vi "SubpanelGuiTemplate.vi"() -> ()   [LabVIEW 2016]
uses:
  <vilib>/Utility/miscctls.llb/LVRowAndColumnUnsignedTypeDef.ctl
  Controls/Messages/DAQControl.ctl
panel:
  in  "Average":bool
  in  "Device":tag
  in  "Add Channel":bool
  in  "Channel":string
  in  "Channel Name":string
  in  "Save Config":bool
  in  "Load Config":bool
  in  "Measurement Rate (Hz)":dbl=2.0
  in  "Average Samples":i32=10
  in  "Stop DAQ":bool
  in  "Start DAQ":bool
  in  "Thermocouple Channels":i32(listbox)
  in  "Remove":bool
  in  "Add":bool
  in  "Control Thermocouple Channels":i32(listbox)
  out "Temperature Profile":cluster{"X":dbl[], "Y":dbl[]}[](graph)
  in  "Name":string="Cycle 1"
  in  "Clear Temps":bool
  in  "Remove Temp":bool
  in  "Add Temp":bool
  in  "Duration":timestamp caption="Duration\n(Hours)" format="%<%H:%M:%S>T"
  in  "Temp":dbl=25.0 caption="Temperature\n(Celsius)"
  in  "Temp Profile List":i32(listbox)=-1
  in  "SaveProfile":bool
  in  "LoadProfile":bool
  in  "Operational Low":dbl=-35.0
  in  "Operational High":dbl=65.0
  in  "Survival Low":dbl=-40.0
  in  "Survival High":dbl=70.0
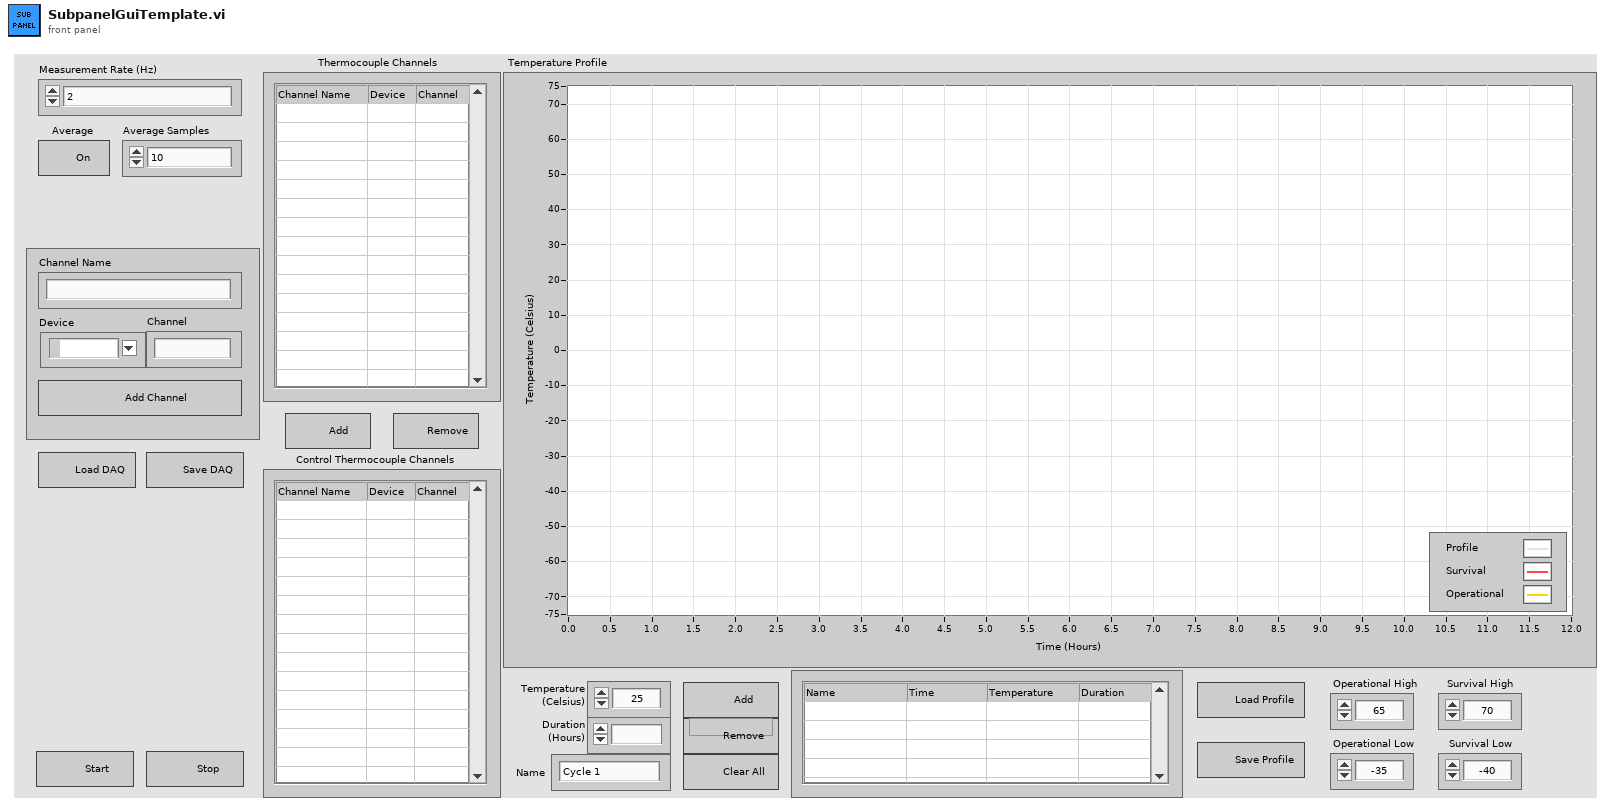
[diagram p1: front panel]
types:
  T1 = typedef "LVRowAndColumnUnsignedTypeDef.ctl" = cluster{"Row":u32, "Column":u32}
  T2 = cluster{"Error":errorcluster, "ChannelList":cluster{"Name":string, "Device":tag, "Channel":string}[], "SampleFreq":dbl, "AvgSamples":i32, "Average":bool, "SampleRate":dbl, "MaxHours":dbl, "TempProfile":dbl[][], "DurationString":string[], "Profile":cluster{"Name":string, "Temperature":string, "Duration":dbl, "Survival High":dbl, "Operational High":dbl, "Operational Low":dbl, "Survival Low":dbl}[], "TempProfileName":string[]}
  T3 = cluster{"Name":string, "Device":tag, "Channel":string}[]
  T4 = cluster{"Name":string, "Device":tag, "Channel":string}
  T5 = typedef "DAQControl.ctl" = cluster{"Timestamp":string, "Timestamp In Seconds":dbl, "DAQ Settings":cluster{"Frequency":dbl, "Averaging":bool, "Average Samples":i32}, "TC Channels":cluster{"Name":string, "Device":string, "Channel":string}[], "Control TCs":string[], "Profile":cluster{"Name":string, "Duration":string, "Temperature":dbl, "Survival High":dbl, "Operational High":dbl, "Operational Low":dbl, "Survival Low":dbl}[], "State":bool}
  T6 = typedef "LVRectTypeDef.ctl" = cluster{"Left":i16, "Top":i16, "Right":i16, "Bottom":i16}
  T7 = cluster{"Channel Name":string, "Device":tag, "Channel":string}
  T8 = cluster{"Channel Name":string, "Device":tag, "Channel":string}[]
  T9 = cluster{"Name":string, "Temperature":string, "Duration":dbl, "Survival High":dbl, "Operational High":dbl, "Operational Low":dbl, "Survival Low":dbl}[]
  T10 = cluster{"SampleFreq":dbl, "Average":bool, "AvgSamples":i32}
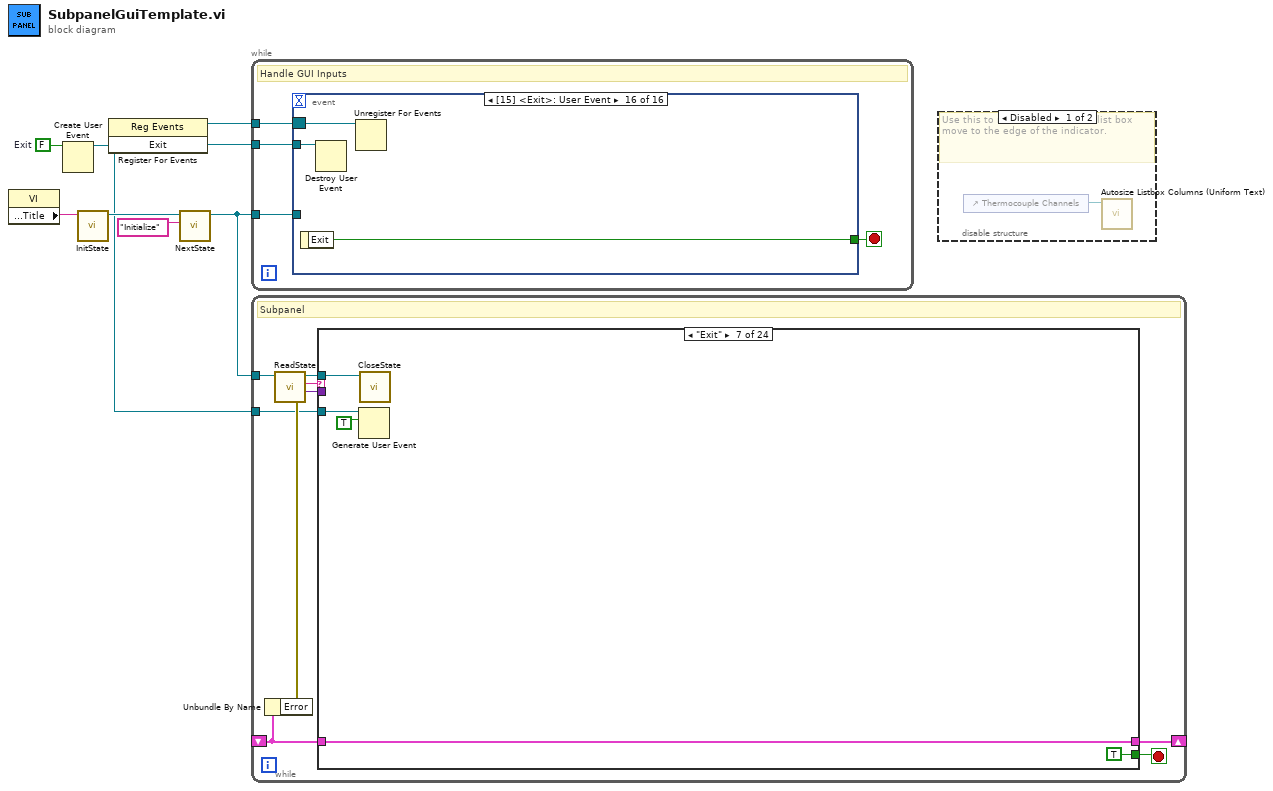
[diagram p0: block diagram]
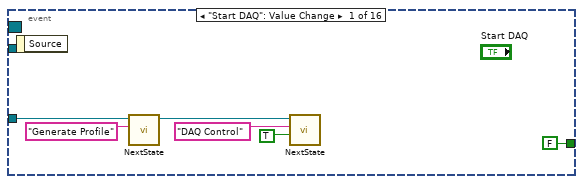
[diagram p3: hidden frame]
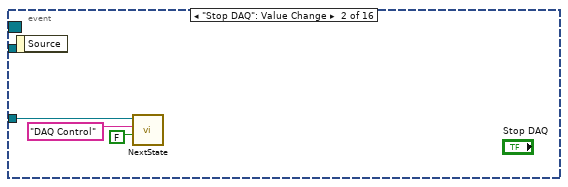
[diagram p4: hidden frame]
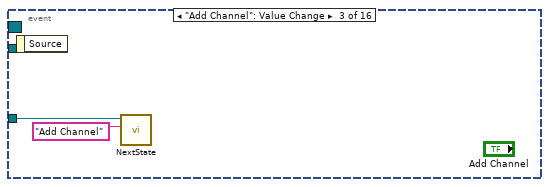
[diagram p5: hidden frame]
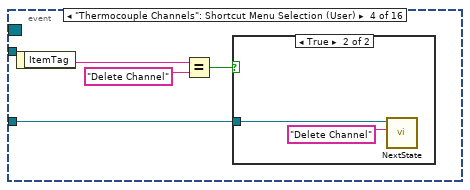
[diagram p6: hidden frame]
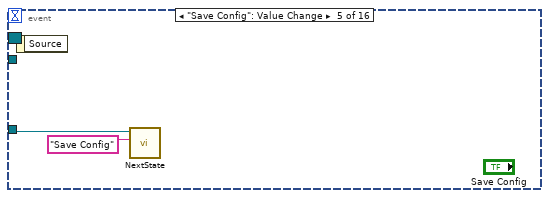
[diagram p8: hidden frame]
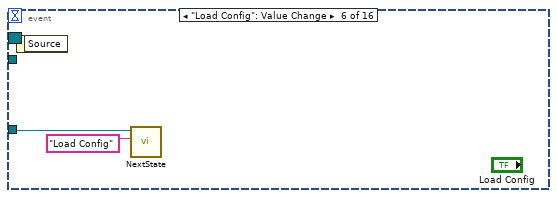
[diagram p9: hidden frame]
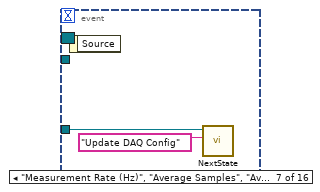
[diagram p10: hidden frame]
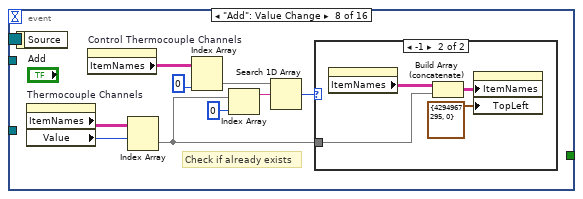
[diagram p11: hidden frame]
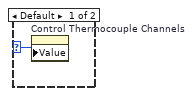
[diagram p12: hidden frame]
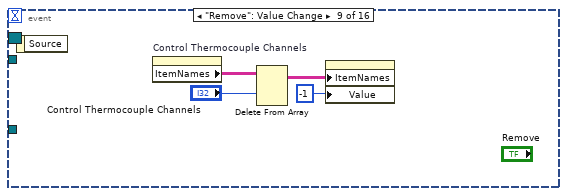
[diagram p13: hidden frame]
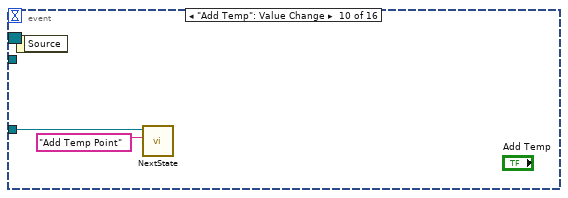
[diagram p14: hidden frame]
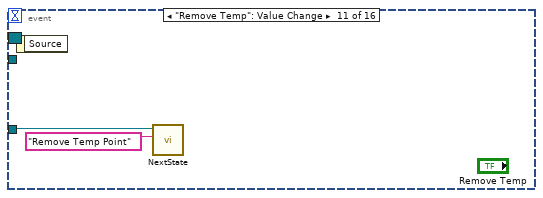
[diagram p15: hidden frame]
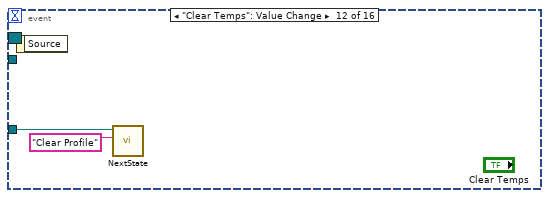
[diagram p16: hidden frame]
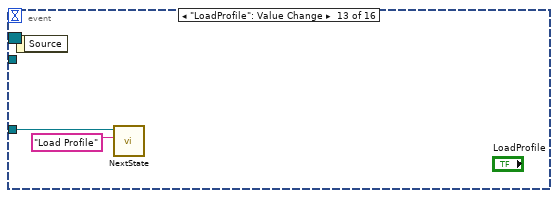
[diagram p17: hidden frame]
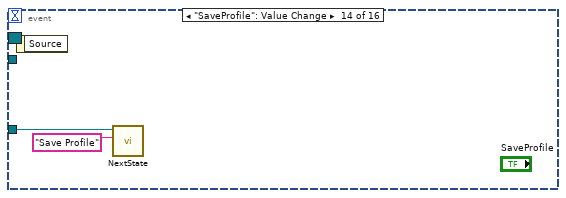
[diagram p18: hidden frame]
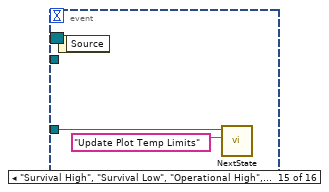
[diagram p19: hidden frame]
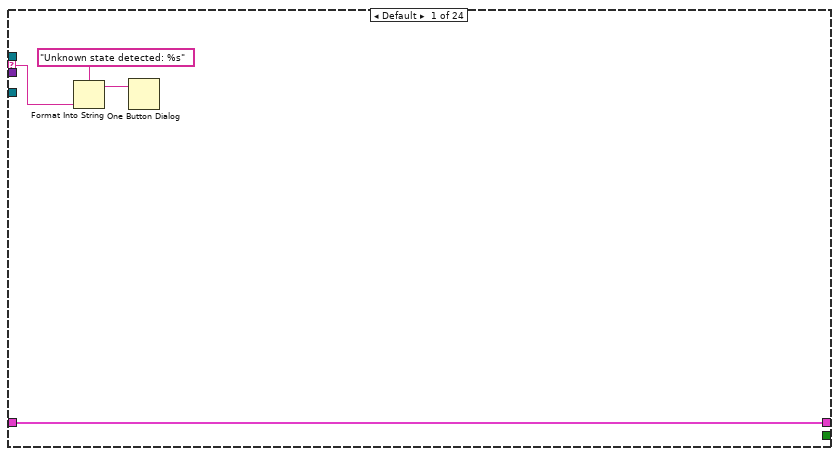
[diagram p20: hidden frame]
diagram:
  w3 = FALSE  # Exit
  n1 = property class="VI"() -> ("Front Panel.Title"=w4:string)  [unwired: 2 in, 2 out]
  n2 = Create User Event(user event datatype=w3) -> (user event=w1:refnum<user-event>)  [unwired: 1 in, 1 out]
  n3 = call "InitState.vi"("Name"=w4) -> ("Queue Out"=w7:refnum<queue>)  [unwired: 8 in, 1 out]
  n4 = register-events(w1) -> (reference out=w2:refnum<event-registration>)  [unwired: 2 in, 1 out]
  n5 = call "NextState.vi"("State"="Initialize" ("element"), "Queue In"=w7) -> ("Queue Out"=w5:refnum<queue>)  [unwired: 8 in, 1 out]
  n6 = while {
    tunnel: w5 -> [w11]
    tunnel: w2 -> [w9]
    tunnel: w1 -> [w8]
    stop <- w10 stop-if-true
    # "Handle GUI Inputs"
    n7 = event shown="[15] <Exit>: User Event" {
      selector: w9 -> [_ _ _ _ _ _ _ _ _ _ _ _ _ _ _ w67]
      dyn-events: _ -> [_ _ _ _ _ _ _ _ _ _ _ _ _ _ _ _]
      timeout: _ -> [_ _ _ _ _ _ _ _ _ _ _ _ _ _ _ _]
      tunnel: w11 -> [w15 w20 w21 w23 w29 w31 w34 _ _ w53 w56 w58 w59 w61 w63 _]
      tunnel: [FALSE _ _ _ _ _ _ _ _ _ _ _ _ _ _ w66] -> w10
      tunnel: w8 -> [_ _ _ _ _ _ _ _ _ _ _ _ _ _ _ w65]
      event "Start DAQ": Value Change {
        n8 = event-data() -> ()  [unwired: 1 in, 1 out]
        n9 = call "NextState.vi"("State"="Generate Profile" ("element"), "Queue In"=w15) -> ("Queue Out"=w14:refnum<queue>)  [unwired: 8 in, 1 out]
        n10 = call "NextState.vi"("Data"=TRUE, "State"="DAQ Control" ("element"), "Queue In"=w14) -> ()  [unwired: 7 in, 2 out]
      }
      event "Stop DAQ": Value Change {
        n11 = event-data() -> ()  [unwired: 1 in, 1 out]
        n12 = call "NextState.vi"("Data"=FALSE, "State"="DAQ Control" ("element"), "Queue In"=w20) -> ()  [unwired: 7 in, 2 out]
      }
      event "Add Channel": Value Change {
        n13 = event-data() -> ()  [unwired: 1 in, 1 out]
        n14 = call "NextState.vi"("State"="Add Channel" ("element"), "Queue In"=w21) -> ()  [unwired: 8 in, 2 out]
      }
      event "Thermocouple Channels": Shortcut Menu Selection (User) {
        n15 = event-data() -> ("ItemTag"=w26:string)  [unwired: 1 in]
        n16 = Equal?(x=w26, y="Delete Channel") -> (x = y?=w24:bool)
        n17 = case shown="True" w24 {
          tunnel: w23 -> [_ w27]
          frame False {
          }
          frame True {
            n18 = call "NextState.vi"("State"="Delete Channel" ("element"), "Queue In"=w27) -> ()  [unwired: 8 in, 2 out]
          }
        }
      }
      event "Save Config": Value Change {
        n19 = event-data() -> ()  [unwired: 1 in, 1 out]
        n20 = call "NextState.vi"("State"="Save Config" ("element"), "Queue In"=w29) -> ()  [unwired: 8 in, 2 out]
      }
      event "Load Config": Value Change {
        n21 = event-data() -> ()  [unwired: 1 in, 1 out]
        n22 = call "NextState.vi"("State"="Load Config" ("element"), "Queue In"=w31) -> ()  [unwired: 8 in, 2 out]
      }
      event "Measurement Rate (Hz)", "Average Samples", "Average": Value Change {
        n23 = event-data() -> ()  [unwired: 1 in, 1 out]
        n24 = call "NextState.vi"("State"="Update DAQ Config" ("element"), "Queue In"=w34) -> ()  [unwired: 8 in, 2 out]
      }
      event "Add": Value Change {
        # "Check if already exists"
        n25 = event-data() -> ()  [unwired: 1 in, 1 out]
        n26 = property on="Thermocouple Channels" class="MCListbox (strict)"() -> ("ItemNames"=w43:string[][], "Value"=w42:i32)  [unwired: 2 in, 2 out]
        n27 = property on="Control Thermocouple Channels" class="MCListbox (strict)"() -> ("ItemNames"=w41:string[][])  [unwired: 2 in, 2 out]
        n28 = Index Array(array=w43, index (row)=w42) -> (element=w35:string[])  [unwired: 1 in]
        n29 = Index Array(array=w41, index (col)=0 ("disabled index (col)")) -> (element=w37:string[])  [unwired: 1 in]
        n30 = Index Array(array=w35, index=0) -> (element=w38:string)
        n31 = Search 1D Array(1D array=w37, element=w38) -> (index of element=w36:i32)  [unwired: 1 in]
        n32 = case shown="-1" w36 {
          selector: w36 -> [w44 _]
          tunnel: w35 -> [_ w46]
          frame Default {
            n33 = property on="Control Thermocouple Channels" class="MCListbox (strict)"("Value"=w44) -> ()  [unwired: 2 in, 2 out]
          }
          frame -1 {
            n34 = property on="Control Thermocouple Channels" class="MCListbox (strict)"() -> ("ItemNames"=w48:string[][])  [unwired: 2 in, 2 out]
            n35 = Build Array (concatenate)(w48, w46) -> (w47:string[][])
            n36 = property on="Control Thermocouple Channels" class="MCListbox (strict)"("ItemNames"=w47, "TopLeft"=T1 {"Row"=4294967295, "Column"=0} ("Top Left Visible Cell")) -> ()  [unwired: 2 in, 2 out]
          }
        }
      }
      event "Remove": Value Change {
        n37 = event-data() -> ()  [unwired: 1 in, 1 out]
        n38 = property on="Control Thermocouple Channels" class="MCListbox (strict)"() -> ("ItemNames"=w52:string[][])  [unwired: 2 in, 2 out]
        n39 = Delete From Array(array=w52, index (row)="Control Thermocouple Channels") -> (array with subset deleted=w51:string[][])  [unwired: 2 in, 1 out]
        n40 = property on="Control Thermocouple Channels" class="MCListbox (strict)"("ItemNames"=w51, "Value"=-1 ("Control Thermocouple Channels")) -> ()  [unwired: 2 in, 2 out]
      }
      event "Add Temp": Value Change {
        n41 = event-data() -> ()  [unwired: 1 in, 1 out]
        n42 = call "NextState.vi"("State"="Add Temp Point" ("element"), "Queue In"=w53) -> ()  [unwired: 8 in, 2 out]
      }
      event "Remove Temp": Value Change {
        n43 = event-data() -> ()  [unwired: 1 in, 1 out]
        n44 = call "NextState.vi"("State"="Remove Temp Point" ("element"), "Queue In"=w56) -> ()  [unwired: 8 in, 2 out]
      }
      event "Clear Temps": Value Change {
        n45 = event-data() -> ()  [unwired: 1 in, 1 out]
        n46 = call "NextState.vi"("State"="Clear Profile" ("element"), "Queue In"=w58) -> ()  [unwired: 8 in, 2 out]
      }
      event "LoadProfile": Value Change {
        n47 = event-data() -> ()  [unwired: 1 in, 1 out]
        n48 = call "NextState.vi"("State"="Load Profile" ("element"), "Queue In"=w59) -> ()  [unwired: 8 in, 2 out]
      }
      event "SaveProfile": Value Change {
        n49 = event-data() -> ()  [unwired: 1 in, 1 out]
        n50 = call "NextState.vi"("State"="Save Profile" ("element"), "Queue In"=w61) -> ()  [unwired: 8 in, 2 out]
      }
      event "Survival High", "Survival Low", "Operational High", "Operational Low": Value Change {
        n51 = event-data() -> ()  [unwired: 1 in, 1 out]
        n52 = call "NextState.vi"("State"="Update Plot Temp Limits" ("element"), "Queue In"=w63) -> ()  [unwired: 8 in, 2 out]
      }
      event User Event {
        n53 = event-data() -> ("Exit"=w66:bool)  [unwired: 1 in]
        n54 = Destroy User Event(user event=w65) -> ()  [unwired: 1 in, 1 out]
        n55 = Unregister For Events(event registration refnum=w67) -> ()  [unwired: 1 in, 1 out]
      }
    }
  }
  n56 = while {
    tunnel: w5 -> [w74]
    shift-right: [w76] -> _
    shift-left: _ -> [w70]
    tunnel: w1 -> [w68]
    stop <- w75 stop-if-true
    # "Subpanel"
    n57 = Unbundle By Name(w70) -> ("Error"=w69:errorcluster)
    n58 = call "ReadState.vi"("Error In"=w69, "Queue In"=w74) -> ("Data"=w71:variant, "State"=w72:string, "Queue Out"=w73:refnum<queue>)  [unwired: 6 in, 1 out]
    n59 = case shown="\"Exit\"" w72 {
      tunnel: w71 -> [_ _ _ _ w112 _ _ _ _ _ _ _ _ w192 _ _ _ _ _ _ _ w358 _ w413]
      selector: w72 -> [w79 _ _ _ _ _ _ _ _ _ _ _ _ _ _ _ _ _ _ _ w319 _ _ _]
      tunnel: [w77 w81 T2 {"Error"={"status"=FALSE, "code"=0, "source"=""}, "ChannelList"=[], "SampleFreq"=2.0, "AvgSamples"=10, "Average"=FALSE, "SampleRate"=0.0, "MaxHours"=12.0, "TempProfile"=[], "DurationString"=[], "Profile"=[], "TempProfileName"=[]} w108 w109 w116 w121 w123 w127 w135 w147 w158 w164 w195 w233 w250 w261 w275 w283 w287 w317 w369 w404 w423] -> w76
      tunnel: [_ _ _ _ _ _ TRUE _ _ _ _ _ _ _ _ _ _ _ _ _ _ _ _ _] -> w75
      tunnel: w70 -> [w77 w81 _ w108 w109 w115 w121 w123 w128 w136 w147 w159 w165 w196 w233 w250 w262 w276 w284 w286 w318 w370 w404 w408]
      tunnel: w73 -> [_ _ w97 _ _ w114 w118 _ w124 w139 w145 _ _ w193 _ _ w260 w273 w281 w298 _ w372 _ _]
      tunnel: w68 -> [_ _ _ _ _ _ w120 _ _ _ _ _ _ _ _ _ _ _ _ _ _ _ _ _]
      frame Default {
        n60 = Format Into String(format string="Unknown state detected: %s", w79) -> (resulting string=w78:string)  [unwired: 2 in, 1 out]
        n61 = One Button Dialog(message=w78) -> ()  [unwired: 1 in, 1 out]
      }
      frame "--- System ---" {
      }
      frame "Initialize" {
        w92 = string[][] [] ("Item Names")
        n62 = call "NextState.vi"("State"="Size Panel" ("element"), "Queue In"=w97) -> ("Queue Out"=w88:refnum<queue>)  [unwired: 8 in, 1 out]
        n63 = call <vilib>:"Application Directory.vi"() -> ("Application Directory"=w95:path)
        n64 = Build Path(base path=w95, name or relative path="Config\\DefaultConfig.csv") -> (appended path=w93:path)
        n65 = call "NextState.vi"("Data"=w93, "State"="Load Config" ("element"), "Queue In"=w88) -> ("Queue Out"=w84:refnum<queue>)  [unwired: 7 in, 1 out]
        n66 = call <vilib>:"Application Directory.vi"() -> ("Application Directory"=w85:path)
        n67 = Build Path(base path=w85, name or relative path="Config\\DefaultProfile.csv") -> (appended path=w87:path)
        n68 = property on="Temp Profile List" class="MCListbox (strict)"("ItemNames"=string[][] [] ("Item Names"), "Value"=-1 ("Temp Profile List")) -> ()  [unwired: 2 in, 2 out]
        n69 = property on="Thermocouple Channels" class="MCListbox (strict)"("ItemNames"=w92) -> ()  [unwired: 2 in, 2 out]
        n70 = property on="Control Thermocouple Channels" class="MCListbox (strict)"("ItemNames"=w92) -> ()  [unwired: 2 in, 2 out]
        n71 = call "NextState.vi"("Data"=w87, "State"="Load Profile" ("element"), "Queue In"=w84) -> ()  [unwired: 7 in, 2 out]
        n72 = property on="Temperature Profile" class="XYGraph (strict)"("Value"=cluster{"X":dbl[], "Y":dbl[]}[] [{"X"=[0.0, 12.0], "Y"=[0.0, 0.0]}, {"X"=[0.0, 12.0], "Y"=[0.0, 0.0]}, {"X"=[0.0, 12.0], "Y"=[0.0, 0.0]}, {"X"=[0.0, 12.0], "Y"=[0.0, 0.0]}, {"X"=[0.0, 12.0], "Y"=[0.0, 0.0]}]) -> ()  [unwired: 2 in, 2 out]
      }
      frame "Size Panel" {
        n73 = property class="VI"() -> ("Front Panel.PanelBounds"=w102:T6)  [unwired: 2 in, 2 out]
        n74 = Unbundle By Name(w102) -> ("Right"=w106:i16, "Left"=w107:i16)
        n75 = Subtract(x=w106, y=w107) -> (x-y=w101:i16)
        n76 = Subtract(x=w101, y=i16 405) -> (x-y=w99:i16)
        n77 = Bundle(0, 2) -> (w103:cluster{i32, i32})  [unwired: 1 in]
        n78 = property on="Thermocouple Channels" class="MCListbox (strict)"("ActiveCell"=w103, "Width"=w99) -> ()  [unwired: 2 in, 2 out]
      }
      frame "Wait" {
        n79 = Variant To Data(type=0.0, Variant=w112) -> (data=w110:dbl)  [unwired: 1 in, 1 out]
        n80 = call "Time Delay"("Delay Time (s)"=w110) -> ()  [unwired: 10 in, 1 out]
      }
      frame "Error" {
        n81 = call "FlushState.vi"("Queue In"=w114) -> ()  [unwired: 9 in, 2 out]
        n82 = Unbundle By Name(w115) -> ("Error"=w117:errorcluster)
        n83 = call <vilib>:"Simple Error Handler.vi"("error in (no error)"=w117) -> ()  [unwired: 4 in, 5 out]
        n84 = Bundle By Name(cluster=w115, "Error"=errorcluster {"status"=FALSE, "code"=0, "source"=""}) -> (w116:T2)
      }
      frame "Exit" {
        n85 = Generate User Event(user event=w120, event data cluster=TRUE ("event data")) -> ()  [unwired: 2 in, 2 out]
        n86 = call "CloseState.vi"("Queue In"=w118) -> ()  [unwired: 10 in, 1 out]
      }
      frame "--- DAQ Setup ---" {
      }
      frame "Add Channel" {
        n87 = Unbundle By Name(w128) -> ("ChannelList"=w133:T3)
        n88 = call "NextState.vi"("State"="Update Channel List" ("element"), "Queue In"=w124) -> ()  [unwired: 8 in, 2 out]
        n89 = Bundle("Channel Name"="Channel Name", "Device"="Device", "Channel"="Channel") -> (w129:T7)  [unwired: 1 in]
        n90 = Build Array (concatenate)(w133, w129) -> (w126:T8)
        n91 = Bundle By Name(cluster=w128, "ChannelList"=w126) -> (w127:T2)
      }
      frame "Delete Channel" {
        n92 = Unbundle By Name(w136) -> ("ChannelList"=w138:T3)
        n93 = call "NextState.vi"("State"="Update Channel List" ("element"), "Queue In"=w139) -> ()  [unwired: 8 in, 2 out]
        n94 = Delete From Array(array=w138, index="Thermocouple Channels") -> (array with subset deleted=w134:T3)  [unwired: 1 in, 1 out]
        n95 = Bundle By Name(cluster=w136, "ChannelList"=w134) -> (w135:T2)
      }
      frame "Update Channel List" {
        n96 = Unbundle By Name(w147) -> ("ChannelList"=w141:T3)
        n97 = call "NextState.vi"("State"="Size Panel" ("element"), "Queue In"=w145) -> ()  [unwired: 8 in, 2 out]
        n98 = for {
          tunnel: w141 -> [w152] mode=indexing
          tunnel: [w148] -> w144 mode=indexing
          n99 = Unbundle By Name(w152) -> ("Name"=w150:string, "Device"=w151:tag, "Channel"=w149:string)
          n100 = Build Array(w150, w151, w149) -> (w148:string[])
        }
        n101 = control-ref of="Thermocouple Channels"() -> (w143:refnum<vi>)
        n102 = property on="Thermocouple Channels" class="MCListbox (strict)"("ItemNames"=w144) -> (error out=w142:errorcluster)  [unwired: 2 in, 1 out]
        n103 = call "Autosize Listbox Columns (Uniform Text).vi"("error in (no error)"=w142, "Table Ref"=w143) -> ()  [unwired: 5 in, 1 out]
      }
      frame "Update DAQ Config" {
        n104 = To Double Precision Float(number="Average Samples") -> (double precision float=w153:dbl)
        n105 = Compound Arithmetic op=MULTIPLY("Measurement Rate (Hz)", w153) -> (w156:dbl)
        n106 = Bundle By Name(cluster=w159, "Average"="Average", "SampleFreq"="Measurement Rate (Hz)", "AvgSamples"="Average Samples", "SampleRate"=w156) -> (w158:T2)
      }
      frame "Save Config" {
        n107 = call <vilib>:"Application Directory.vi"() -> ("Application Directory"=w163:path)
        n108 = Build Path(base path=w163, name or relative path="Config") -> (appended path=w160:path)
        n109 = call "File Dialog"("start path"=w160, "default name"="DefaultConfig.csv" ("name or relative path"), "pattern (all files)"="*.csv") -> ("selected path"=w166:path, "cancelled"=w167:bool)  [unwired: 9 in, 2 out]
        n110 = case shown="False" w167 {
          tunnel: w165 -> [w178 _]
          tunnel: w166 -> [w177 _]
          tunnel: w165 -> [w176 w188]
          tunnel: [w175 w188] -> w164
          tunnel: w160 -> [w171 _]
          frame False {
            n111 = Unbundle By Name(w178) -> ("ChannelList"=w180:T3)
            n112 = for {
              tunnel: w180 -> [w187] mode=indexing
              shift-right: [w181] -> w172
              shift-left: "Name,Device,Channel\n" -> [w186]
              n113 = Unbundle By Name(w187) -> ("Name"=w184:string, "Device"=w183:tag, "Channel"=w182:string)
              n114 = Format Into String(format string="%s,%s,%s\n", initial string=w186, w184, w183, w182) -> (resulting string=w181:string)  [unwired: 1 in, 1 out]
            }
            n115 = Write to Text File(file (use dialog)=w177, text=w172) -> (error out=w173:errorcluster)  [unwired: 2 in, 2 out]
            n116 = Build Path(base path=w171, name or relative path="DefaultConfig.csv") -> (appended path=w169:path)
            n117 = Write to Text File(file (use dialog)=w169, text=w172, error in=w173) -> (error out=w174:errorcluster)  [unwired: 1 in, 2 out]
            n118 = Bundle By Name(cluster=w176, "Error"=w174) -> (w175:T2)
          }
          frame True {
          }
        }
      }
      frame "Load Config" {
        n119 = Variant To Data(type=path "" ("selected path"), Variant=w192) -> (data=w189:path)  [unwired: 1 in, 1 out]
        n120 = Empty String/Path?(string/path=w189) -> (empty?=w190:bool)
        n121 = case shown="True" w190 {
          tunnel: [w198 w201] -> w197
          tunnel: [_ w200] -> w194
          tunnel: w189 -> [w198 _]
          frame False {
          }
          frame True {
            n122 = call <vilib>:"Application Directory.vi"() -> ("Application Directory"=w205:path)
            n123 = Build Path(base path=w205, name or relative path="Config") -> (appended path=w203:path)
            n124 = call "File Dialog2"("start path"=w203, "default name"="DefaultConfig.csv" ("name or relative path"), "pattern (all files)"="*.csv") -> ("selected path"=w201:path, "cancelled"=w200:bool)  [unwired: 9 in, 2 out]
          }
        }
        n125 = case shown="False" w194 {
          tunnel: w197 -> [w217 _]
          tunnel: w196 -> [w210 w232]
          tunnel: [w208 w232] -> w195
          tunnel: w193 -> [w206 _]
          frame False {
            n126 = Read from Text File(file (use dialog)=w217) -> (text=w216:string)  [unwired: 3 in, 3 out]
            n127 = Spreadsheet String To Array(delimiter (Tab)=",", format string="%s", spreadsheet string=w216, array type (2D Dbl)=string[][] []) -> (array=w212:string[][])
            n128 = call "NextState.vi"("State"="Update Channel List" ("element"), "Queue In"=w206) -> ()  [unwired: 8 in, 2 out]
            n129 = for {
              tunnel: w212 -> [w227] mode=indexing
              shift-right: [w220] -> w209
              shift-left: T3 [] ("ChannelList") -> [w224]
              i -> [w223]
              n130 = Index Array(array=w227) -> (element #1=w222:string, element #2=w226:string, element #3=w225:string)  [unwired: 3 in]
              n131 = Equal To 0?(x=w223) -> (x = 0?=w219:bool)
              n132 = Bundle By Name(cluster=T4 {"Name"="", "Device"="", "Channel"=""} ("ChannelDefinition"), "Name"=w222, "Device"=w226, "Channel"=w225) -> (w218:T4)
              n133 = case shown="False" w219 {
                tunnel: w224 -> [w230 w231]
                tunnel: [w229 w231] -> w220
                tunnel: w218 -> [w228 _]
                frame False {
                  n134 = Build Array (concatenate)(w230, w228) -> (w229:T3)
                }
                frame True {
                }
              }
            }
            n135 = Bundle By Name(cluster=w210, "ChannelList"=w209) -> (w208:T2)
          }
          frame True {
          }
        }
      }
      frame "--- Setup Temp Profile ---" {
      }
      frame "Update Plot Temp Limits" {
        n136 = property on="Temperature Profile" class="XYGraph (strict)"() -> ("Value"=w246:cluster{"X":dbl[], "Y":dbl[]}[])  [unwired: 2 in, 2 out]
        n137 = Index Array(array=w246) -> (element=w249:cluster{"X":dbl[], "Y":dbl[]})  [unwired: 1 in]
        n138 = Unbundle By Name(w249) -> ("X"=w240:dbl[])
        n139 = Build Array("Survival High", "Operational High", "Operational Low", "Survival Low") -> (w239:dbl[])
        n140 = Array Size(array=w240) -> (size(s)=w247:i32)
        n141 = for {
          tunnel: w239 -> [w255] mode=indexing
          tunnel: w247 -> [w254]
          tunnel: [w253] -> w248 mode=indexing
          tunnel: w240 -> [w252]
          n142 = Initialize Array(w255, w254) -> (w251:dbl[])
          n143 = Bundle("X"=w252, w251) -> (w253:cluster{"X":dbl[], dbl[]})  [unwired: 1 in]
        }
        n144 = Absolute Value(x=w239) -> (abs(x)=w238:dbl[])
        n145 = Array Max & Min(array=w238) -> (max value=w236:dbl)  [unwired: 3 out]
        n146 = Add(x=w236, y=5.0) -> (x+y=w234:dbl)
        n147 = Build Array (concatenate)(w249, w248) -> (w241:cluster{"X":dbl[], "Y":dbl[]}[])
        n148 = Negate(x=w234) -> (-x=w237:dbl)
        n149 = property on="Temperature Profile" class="XYGraph (strict)"("Value"=w241, "YScale.Minimum"=w237, "YScale.Maximum"=w234) -> ()  [unwired: 2 in, 2 out]
      }
      frame "Add Temp Point" {
        n150 = Unbundle By Name(w262) -> ("TempProfileName"=w258:string[], "TempProfile"=w265:dbl[][])
        n151 = call "NextState.vi"("State"="Update Profile" ("element"), "Queue In"=w260) -> ()  [unwired: 8 in, 2 out]
        n152 = Subtract(x="Duration", y=timestamp(-57600 s since 1904-01-01)) -> (x-y=w267:dbl)
        n153 = Build Array(w267, "Temp") -> (w264:dbl[])
        n154 = Build Array (concatenate)(w258, "Name") -> (w256:string[])
        n155 = Build Array (concatenate)(w265, w264) -> (w263:dbl[][])
        n156 = Bundle By Name(cluster=w262, "TempProfileName"=w256, "TempProfile"=w263) -> (w261:T2)
      }
      frame "Remove Temp Point" {
        n157 = Unbundle By Name(w276) -> ("TempProfileName"=w272:string[], "TempProfile"=w278:dbl[][])
        n158 = call "NextState.vi"("State"="Update Profile" ("element"), "Queue In"=w273) -> ()  [unwired: 8 in, 2 out]
        n159 = Delete From Array(array=w272, index="Temp Profile List") -> (array with subset deleted=w270:string[])  [unwired: 1 in, 1 out]
        n160 = Delete From Array(array=w278, index (row)="Temp Profile List") -> (array with subset deleted=w277:dbl[][])  [unwired: 2 in, 1 out]
        n161 = Bundle By Name(cluster=w276, "TempProfileName"=w270, "TempProfile"=w277) -> (w275:T2)
      }
      frame "Clear Profile" {
        n162 = call "NextState.vi"("State"="Update Profile" ("element"), "Queue In"=w281) -> ()  [unwired: 8 in, 2 out]
        n163 = Bundle By Name(cluster=w284, "TempProfileName"=string[] [], "TempProfile"=dbl[][] []) -> (w283:T2)
      }
      frame "Update Profile" {
        w300 = 0.0  # Time
        # "0 = Duration (seconds)\n1 = Temperature (C)"
        n164 = Unbundle By Name(w286) -> ("TempProfileName"=w285:string[])
        n165 = Unbundle By Name(w286) -> ("TempProfile"=w301:dbl[][])
        n166 = call "NextState.vi"("State"="Update Plot Temp Limits" ("element"), "Queue In"=w298) -> ()  [unwired: 8 in, 2 out]
        n167 = for {
          tunnel: w301 -> [w313] mode=indexing
          shift-right: [w305] -> _
          shift-left: w300 -> [w312]
          tunnel: [w306] -> w299 mode=indexing
          tunnel: [w305] -> w292 mode=indexing
          tunnel: [w304] -> w296 mode=indexing
          tunnel: [w303] -> w288 mode=indexing
          tunnel: w285 -> [w302] mode=indexing
          n168 = Index Array(array=w313) -> (element #1=w310:dbl, element #2=w304:dbl)  [unwired: 2 in]
          n169 = Format Into String(format string="%<%H:%M:%S>t", w312) -> (resulting string=w307:string)  [unwired: 2 in, 1 out]
          n170 = Format Into String(format string="%<%H:%M:%S>t", w310) -> (resulting string=w303:string)  [unwired: 2 in, 1 out]
          n171 = Number To Fractional String(number=w304, precision (6)=i16 1) -> (F-format string=w308:string)  [unwired: 2 in]
          n172 = Compound Arithmetic op=ADD(w312, w310) -> (w305:dbl)
          n173 = Build Array(w302, w307, w308, w303) -> (w306:string[])
        }
        n174 = property on="Temperature Profile" class="XYGraph (strict)"() -> ("Value"=w295:cluster{"X":dbl[], "Y":dbl[]}[])  [unwired: 2 in, 2 out]
        n175 = property on="Temp Profile List" class="MCListbox (strict)"("ItemNames"=w299) -> ()  [unwired: 2 in, 2 out]
        n176 = Bundle By Name(cluster=w286, "DurationString"=w288) -> (w287:T2)
        n177 = Divide(x=w292, y=3600.0 ("result")) -> (x/y=w290:dbl[])
        n178 = Bundle(w290, w296) -> (w293:cluster{dbl[], dbl[]})  [unwired: 1 in]
        n179 = Replace Array Subset(array=w295, new element=w293, index=0) -> (→"Temperature Profile":cluster{"X":dbl[], "Y":dbl[]}[])
      }
      frame "Generate Profile", "Save Profile" {
        # "Name, Duration(HH:MM:SS), Temperature(C), Surv High, Op High, Op Low, Surv Low"
        n180 = Unbundle By Name(w318) -> ("TempProfileName"=w315:string[], "DurationString"=w333:string[])
        n181 = property on="Temperature Profile" class="XYGraph (strict)"() -> ("Value"=w332:cluster{"X":dbl[], "Y":dbl[]}[])  [unwired: 2 in, 2 out]
        n182 = Index Array(array=w332) -> (element #1=w324:cluster{"X":dbl[], "Y":dbl[]}, element #2=w323:cluster{"X":dbl[], "Y":dbl[]}, element #3=w322:cluster{"X":dbl[], "Y":dbl[]}, element #4=w321:cluster{"X":dbl[], "Y":dbl[]}, element #5=w320:cluster{"X":dbl[], "Y":dbl[]})  [unwired: 5 in]
        n183 = Unbundle By Name(w324) -> ("Y"=w329:dbl[])
        n184 = Unbundle By Name(w323) -> ("Y"=w328:dbl[])
        n185 = Unbundle By Name(w322) -> ("Y"=w327:dbl[])
        n186 = Unbundle By Name(w321) -> ("Y"=w326:dbl[])
        n187 = Unbundle By Name(w320) -> ("Y"=w325:dbl[])
        n188 = for {
          tunnel: w333 -> [w347] mode=indexing
          shift-right: [w355] -> w331
          shift-left: "Cycle Name,Duration,Temperature,Surival High,Operational High,Operational Low,Survival Low\n" -> [w356]
          tunnel: w329 -> [w348] mode=indexing
          tunnel: w328 -> [w350] mode=indexing
          tunnel: w327 -> [w351] mode=indexing
          tunnel: w326 -> [w352] mode=indexing
          tunnel: w325 -> [w353] mode=indexing
          tunnel: [w349] -> w316 mode=indexing
          tunnel: w315 -> [w346] mode=indexing
          n189 = Format Into String(format string="%s,%s,%.1f,%.1f,%.1f,%.1f,%.1f\n", initial string=w356, w346, w347, w348, w350, w351, w352, w353) -> (resulting string=w355:string)  [unwired: 1 in, 1 out]
          n190 = Bundle(w346, w347, w348, w350, w351, w352, w353) -> (w349:cluster{string, string, dbl, dbl, dbl, dbl, dbl})  [unwired: 1 in]
        }
        n191 = case shown="\"Generate Profile\"" w319 {
          tunnel: w331 -> [_ w342 _]
          tunnel: w318 -> [w334 w341 w345]
          tunnel: [w334 w341 w344] -> w317
          tunnel: w316 -> [_ _ w343]
          frame Default {
          }
          frame "Save Profile" {
            n192 = call <vilib>:"Application Directory.vi"() -> ("Application Directory"=w340:path)
            n193 = Build Path(base path=w340, name or relative path="Config") -> (appended path=w338:path)
            n194 = call "File Dialog3"("start path"=w338, "default name"="DefaultProfile.csv" ("name or relative path"), "pattern (all files)"="*.csv") -> ("selected path"=w335:path)  [unwired: 9 in, 3 out]
            n195 = Write to Text File(file (use dialog)=w335, text=w342) -> ()  [unwired: 2 in, 3 out]
          }
          frame "Generate Profile" {
            n196 = Bundle By Name(cluster=w345, "Profile"=w343) -> (w344:T2)
          }
        }
      }
      frame "Load Profile" {
        n197 = Variant To Data(type=path "" ("selected path"), Variant=w358) -> (data=w361:path)  [unwired: 1 in, 1 out]
        n198 = Empty String/Path?(string/path=w361) -> (empty?=w360:bool)
        n199 = case shown="True" w360 {
          tunnel: [w373 w375] -> w357
          tunnel: w361 -> [w373 _]
          frame False {
          }
          frame True {
            n200 = call <vilib>:"Application Directory.vi"() -> ("Application Directory"=w379:path)
            n201 = Build Path(base path=w379, name or relative path="Config") -> (appended path=w377:path)
            n202 = call "File Dialog5"("start path"=w377, "default name"="DefaultProfile.csv" ("name or relative path"), "pattern (all files)"="*.csv") -> ("selected path"=w375:path)  [unwired: 9 in, 3 out]
          }
        }
        n203 = Read from Text File(file (use dialog)=w357) -> (text=w368:string)  [unwired: 3 in, 3 out]
        n204 = Spreadsheet String To Array(delimiter (Tab)=",", format string="%s", spreadsheet string=w368, array type (2D Dbl)=string[][] []) -> (array=w364:string[][])
        n205 = for {
          tunnel: w364 -> [w385] mode=indexing
          tunnel: [w387] -> w363 mode=indexing if=w380
          tunnel: [w386] -> w362 mode=indexing if=w380
          i -> [w381]
          n206 = Split 1D Array(array=w385, index=1) -> (first subarray=w383:string[], second subarray=w382:string[])
          n207 = Fract/Exp String To Number(string=w382) -> (number=w389:dbl[])  [unwired: 3 in, 1 out]
          n208 = Index Array(array=w383) -> (element=w386:string)  [unwired: 1 in]
          n209 = Index Array(array=w382) -> (element=w403:string)  [unwired: 1 in]
          n210 = Match Pattern(string=w403, regular expression=":") -> (before substring=w399:string, after substring=w401:string)  [unwired: 1 in, 2 out]
          n211 = Fract/Exp String To Number(string=w399) -> (number=w398:dbl)  [unwired: 3 in, 1 out]
          n212 = Match Pattern(string=w401, regular expression=":") -> (before substring=w396:string, after substring=w395:string)  [unwired: 1 in, 2 out]
          n213 = Fract/Exp String To Number(string=w395) -> (number=w392:dbl)  [unwired: 3 in, 1 out]
          n214 = Compound Arithmetic op=MULTIPLY(3600.0 ("value"), w398) -> (w390:dbl)
          n215 = Fract/Exp String To Number(string=w396) -> (number=w394:dbl)  [unwired: 3 in, 1 out]
          n216 = Compound Arithmetic op=MULTIPLY(60.0 ("value"), w394) -> (w391:dbl)
          n217 = Compound Arithmetic op=ADD(w390, w391, w392) -> (w388:dbl)
          n218 = Not Equal To 0?(x=w381) -> (x != 0?=w380:bool)
          n219 = Replace Array Subset(array=w389, new element=w388) -> (w387:dbl[])  [unwired: 1 in]
        }
        n220 = call "NextState.vi"("State"="Update Profile" ("element"), "Queue In"=w372) -> ()  [unwired: 8 in, 2 out]
        n221 = Bundle By Name(cluster=w370, "TempProfile"=w363, "TempProfileName"=w362) -> (w369:T2)
      }
      frame "--- DAQ Control ---" {
      }
      frame "DAQ Control" {
        n222 = Unbundle By Name(w408) -> ("SampleFreq"=w418:dbl, "Average"=w420:bool, "AvgSamples"=w419:i32)
        n223 = Unbundle By Name(w408) -> ("ChannelList"=w416:T3, "Profile"=w410:T9)
        n224 = Variant To Data(type=FALSE, Variant=w413) -> (data=w411:bool)  [unwired: 1 in, 1 out]
        n225 = Bundle("SampleFreq"=w418, "Average"=w420, "AvgSamples"=w419) -> (w417:T10)  [unwired: 1 in]
        n226 = property on="Control Thermocouple Channels" class="MCListbox (strict)"() -> ("ItemNames"=w415:string[][])  [unwired: 2 in, 2 out]
        n227 = for {
          tunnel: w415 -> [w440] mode=indexing
          tunnel: [w439] -> w414 mode=indexing
          n228 = Index Array(array=w440) -> (element=w439:string)  [unwired: 1 in]
        }
        n229 = Get Date/Time In Seconds() -> (seconds since 1Jan1904=w407:timestamp)
        n230 = Format Date/Time String(seconds (now)=w407) -> (date/time string=w406:string)  [unwired: 2 in]
        n231 = To Double Precision Float(number=w407) -> (double precision float=w405:dbl)
        n232 = disable-structure shown="Disabled" {
          disable-tunnel: [w437 _] -> w424
          disable-tunnel: [w435 _] -> w421
          disable-tunnel: w417 -> [w433 _]
          disable-tunnel: w416 -> [w432 _]
          disable-tunnel: w414 -> [w431 _]
          disable-tunnel: w411 -> [w430 _]
          disable-tunnel: w410 -> [w429 _]
          disable-tunnel: w406 -> [w428 _]
          disable-tunnel: w405 -> [w427 _]
          frame Disabled {
            n233 = Bundle By Name(cluster=T5 {"Timestamp"="", "Timestamp In Seconds"=0.0, "DAQ Settings"={"Frequency"=0.0, "Averaging"=TRUE, "Average Samples"=0}, "TC Channels"=[], "Control TCs"=[], "Profile"=[], "State"=FALSE}, "Timestamp In Seconds"=w427, "Timestamp"=w428, "State"=w430, "DAQ Settings"=w433, "TC Channels"=w432, "Profile"=w429, "Control TCs"=w431) -> (w436:T5)
            n234 = Flatten To JSON(anything=w436) -> (JSON string=w435:string)  [unwired: 2 in, 1 out]
            n235 = call "MessageQueue-PublishMessage.vi"("Message"=w435, "Topic"="DAQ Control") -> ("error out"=w437:errorcluster)  [unwired: 8 in, 1 out]
          }
          frame Enabled {
          }
        }
        n236 = call "InitState.vi"("Name"="MainPanel" ("name (unnamed)")) -> ("Queue Out"=w425:refnum<queue>)  [unwired: 8 in, 1 out]
        n237 = call "WriteToLog.vi"("Error In"=w424, "Data"=w421, "Source"="TC DAQ Settings", "Queue In"=w425) -> ("Error Out"=w409:errorcluster)  [unwired: 6 in, 1 out]
        n238 = Bundle By Name(cluster=w408, "Error"=w409) -> (w423:T2)
      }
    }
  }
  n239 = disable-structure shown="Disabled" {
    frame Disabled {
      # "Use this to make last column in list box move to the edge of the indicator."
      n240 = control-ref of="Thermocouple Channels"() -> (w441:refnum<vi>)
      n241 = call "Autosize Listbox Columns (Uniform Text).vi"("Table Ref"=w441) -> ()  [unwired: 6 in, 1 out]
    }
    frame Enabled {
    }
  }
